vi "ClimbSetSensorPoseLeft.vi"(8 "ClimbSetSensorPoseLeft":dbl) -> ()   [LabVIEW 2023]
uses:
  ClimbGlobal.vi
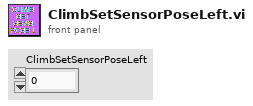
[diagram p1: front panel]
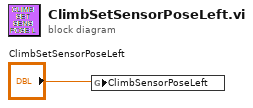
[diagram p0: block diagram]
diagram:
  n1 = global write "ClimbGlobal.vi" "ClimbSensorPoseLeft"("ClimbSetSensorPoseLeft") -> ()
